vi "Refresh Current DQMH Module.vi"(0 "Tree Map In":T2, 1 "DQMH Lib Ref":refnum<vi>, 2 "Modules Type":T1, 3 "App Ref":refnum<vi>, 7 "Project Name":string="Project", 9 "Parent Path":string, 11 "error in":errorcluster, 14 "TreeControl in":refnum<vi>) -> (4 "Tree Map out":T2, 15 "error out":errorcluster)   [LabVIEW 2019, in "Panther Dashboard.lvlib"]
uses:
  Panther Dashboard.lvlib
  <vilib>/National Instruments/Tree Map/Tree Map.lvlib
  <vilib>/National Instruments/Tree Map/Tree Map Data.ctl
  Module type--enum.ctl
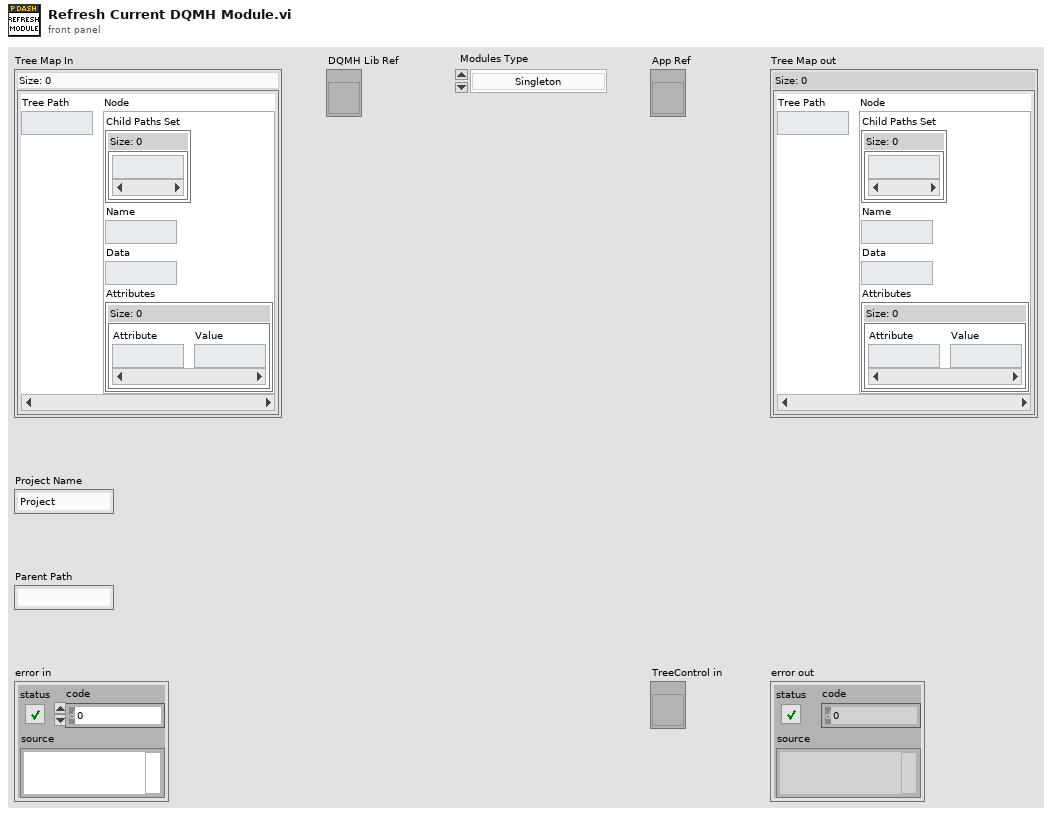
[diagram p1: front panel]
types:
  T1 = typedef "Panther Dashboard.lvlib/Module type--enum.ctl" = enum16{"Singleton", "Cloneable"}
  T2 = typedef "Tree Map.lvlib/Tree Map Data.ctl" = map{string, cluster{"Child Paths Set":set{string}, "Name":string, "Data":string, "Attributes":map{string, string}}}
  T3 = cluster{"Left Cell String":string, "Child Text":string[], "Child Tag":string, "Item Indent":i32, "Child Only?":bool, "Glyph Index":i32}[]
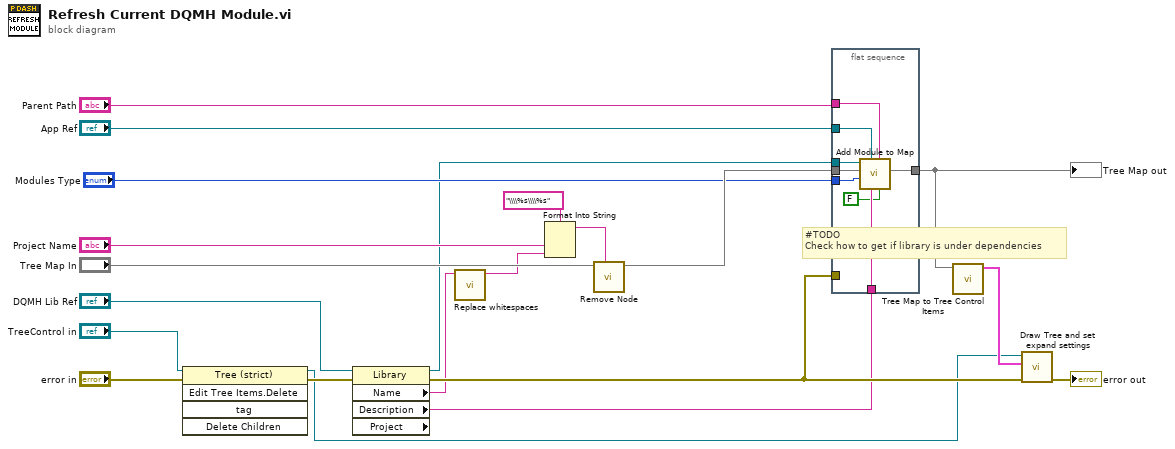
[diagram p0: block diagram]
diagram:
  # "#TODO\nCheck how to get if library is under dependencies"
  n1 = invoke on="Invoke Node" class="Tree (strict)" method="Edit Tree Items.Delete"(reference="TreeControl in", error in="error in") -> (reference out=w9:refnum<vi>, error out=w21:errorcluster)  [unwired: 3 in, 3 out]
  n2 = property class="Library" props=["Name", "Description", "Project"](reference="DQMH Lib Ref", error in=w21) -> (reference out=w1:refnum<vi>, error out=w18:errorcluster, "Name"=w6:string, "Description"=w2:string)  [unwired: 1 out]
  n3 = call "Replace whitespaces.vi"("Text"=w6) -> ("text with spaces replaced"=w4:string)  [unwired: 10 in]
  n4 = Format Into String(format string="\\\\%s\\\\%s", "Project Name", w4) -> (resulting string=w14:string)  [unwired: 2 in, 1 out]
  n5 = call <vilib>:"Remove Node.vi"("Node Path"=w14, "Tree Map In"="Tree Map In") -> ("Tree Map Out"=w11:T2)  [unwired: 7 in, 2 out]
  n6 = flat-sequence {
    tunnel: [w29] -> w13
    tunnel: w11 -> [w28]
    tunnel: "App Ref" -> [w27]
    tunnel: w1 -> [w26]
    tunnel: "Parent Path" -> [w25]
    tunnel: w18 -> [_]
    tunnel: "Modules Type" -> [w24]
    tunnel: w2 -> [w23]
    frame #0 {
      n7 = call "Add Module to Map.vi"("is Dependency?"=FALSE, "Parent Path"=w25, "Module Description"=w23, "App Ref"=w27, "Modules Types"=w24, "Tree Map in"=w28, "Library in"=w26) -> ("Tree Map out"=w29:T2)  [unwired: 3 in, 1 out]
    }
  }
  n8 = call <vilib>:"Tree Map to Tree Control Items.vi"("Tree Map In"=w13) -> ("Tree Control Items"=w16:T3)  [unwired: 10 in]
  n9 = call "Draw Tree and set expand settings.vi"("error in"=w18, "Tree Control Items"=w16, "TreeControl in"=w9) -> ("error out"=→"error out":errorcluster)  [unwired: 8 in]
  "Tree Map out" <- w13
